vi "Draw Stripe Fill.vi"(6 "Stripe Color":u32(colorbox), 7 "Horizontal or Vertical Stripe?":bool, 8 "error in (no error)":errorcluster, 9 "Stripe End":dbl, 10 "Stripe Start":dbl, 11 "Graph Manager in":refnum<class "Graph Manager.lvclass">) -> (0 "error out":errorcluster, 3 "Graph Manager out":refnum<class "Graph Manager.lvclass">)   [LabVIEW 2014, in "Graph Manager.lvclass"]
uses:
  Graph Manager.lvclass
  Graph Manager.lvclass/Graph Manager.ctl
panel:
  # "NOT FINISHED YET!"
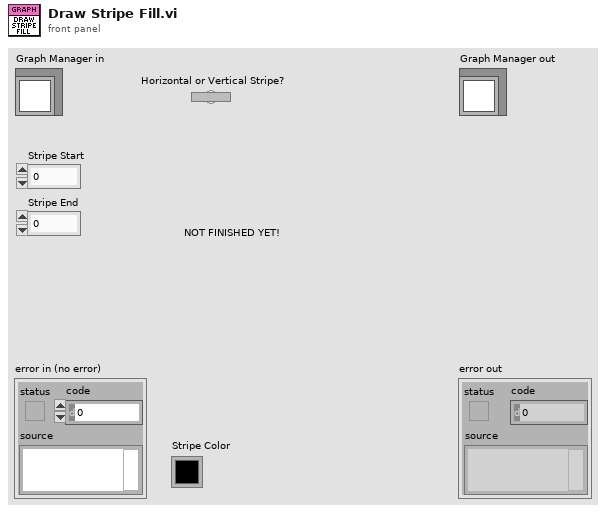
[diagram p1: front panel]
types:
  T1 = cluster{"left":i16, "top":i16, "right":i16, "bottom":i16}
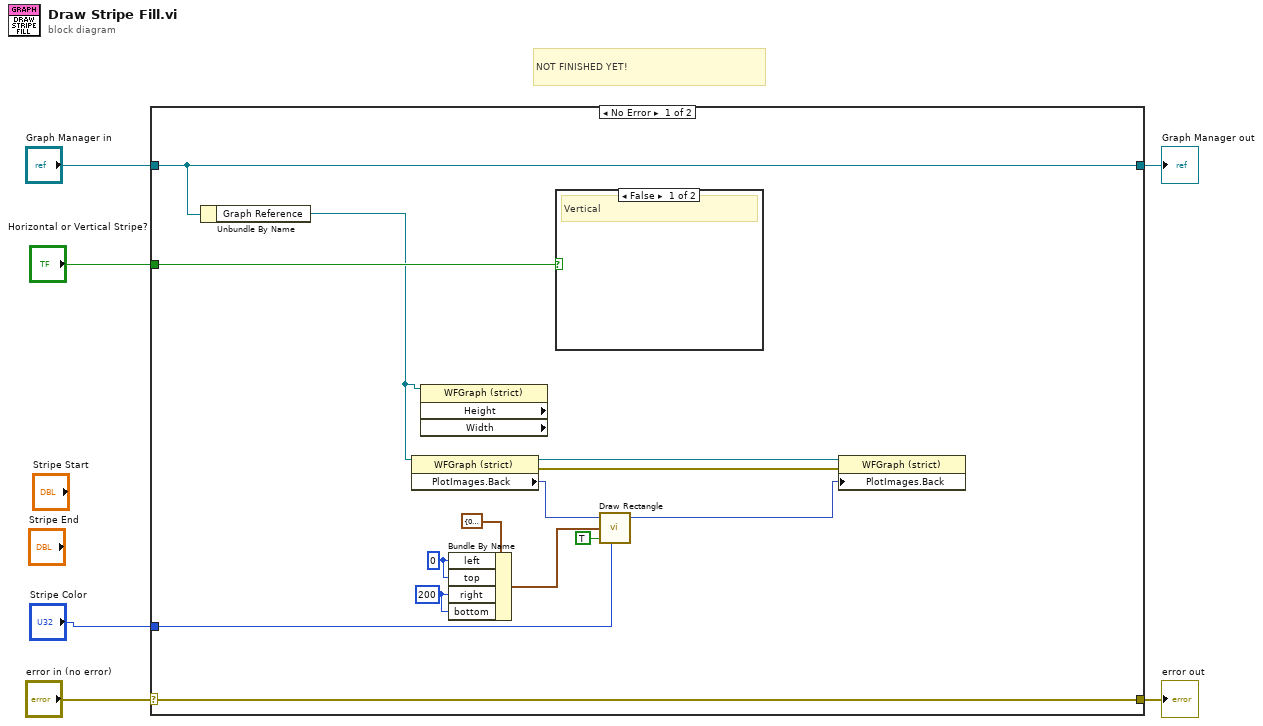
[diagram p0: block diagram]
diagram:
  # "NOT FINISHED YET!"
  n1 = case shown="No Error" "error in (no error)" {
    selector: "error in (no error)" -> [w20 w22]
    tunnel: [w20 w22] -> w5
    tunnel: [w18 w21] -> w3
    tunnel: "Graph Manager in" -> [w18 w21]
    tunnel: "Horizontal or Vertical Stripe?" -> [w19 _]
    tunnel: "Stripe Color" -> [w8 _]
    frame No Error {
      w12 = i16 200 ("right")
      w13 = i16 0 ("left")
      n2 = Unbundle By Name(w18) -> ("Graph Reference"=w11:refnum<vi>)
      n3 = property class="WFGraph (strict)"(reference=w11) -> (reference out=w17:refnum<vi>, error out=w16:errorcluster, "PlotImages.Back"=w15:picture)  [unwired: 1 in]
      n4 = property class="WFGraph (strict)" props=["Height", "Width"](reference=w11) -> ()  [unwired: 1 in, 4 out]
      n5 = Bundle By Name(cluster=T1 {"left"=0, "top"=0, "right"=0, "bottom"=0} ("rect"), "left"=w13, "top"=w13, "right"=w12, "bottom"=w12) -> (w10:T1)
      n6 = case shown="False" w19 {
        frame False {
          # "Vertical"
        }
        frame True {
          # "Horizontal"
        }
      }
      n7 = call <vilib>:"Draw Rectangle.vi"("picture"=w15, "rect"=w10, "fill?(F)"=TRUE, "color(black)"=w8) -> ("new picture"=w7:picture)  [unwired: 5 in]
      n8 = property class="WFGraph (strict)"(reference=w17, error in=w16, "PlotImages.Back"=w7) -> ()  [unwired: 2 out]
    }
    frame Error {
    }
  }
  "error out" <- w5
  "Graph Manager out" <- w3
